vi "Repack Pixels_Pixel Bus to FIFO HSL32x8.vi"(10 "Input Valid":bool=TRUE, 11 "Pixel Bus In":T1={"Pixel Data"={"A"=[0, 0, 0, 0, 0, 0, 0, 0], "R/H"=[0, 0, 0, 0, 0, 0, 0, 0], "G/S"=[0, 0, 0, 0, 0, 0, 0, 0], "B/L"=[0, 0, 0, 0, 0, 0, 0, 0]}, "DV"=[FALSE, FALSE, FALSE, FALSE, FALSE, FALSE, FALSE, FALSE], "EOL"=FALSE, "EOI"=FALSE, "Data Type"=enum."HSL32 x 8"}) -> (2 "Output Valid":bool, 3 "output array":u32[](array[numeric]))   [LabVIEW 2017, in "NI_VDM_FPGA_Basics.lvlib"]
uses:
  <vilib>/visionFPGA/NI_VDM_FPGA_Basics.lvlib
  <vilib>/visionFPGA/Controls/IMAQ FPGA Pixel Bus HSL32x8.ctl
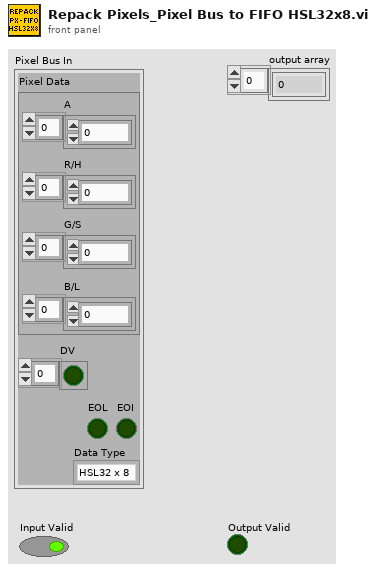
[diagram p1: front panel]
types:
  T1 = typedef "IMAQ FPGA Pixel Bus HSL32x8.ctl" = cluster{"Pixel Data":cluster{"A":u8[], "R/H":u8[], "G/S":u8[], "B/L":u8[]}, "DV":bool[], "EOL":bool, "EOI":bool, "Data Type":enum16{"HSL32 x 8"}}
  T2 = cluster{"A":u8[], "R/H":u8[], "G/S":u8[], "B/L":u8[]}
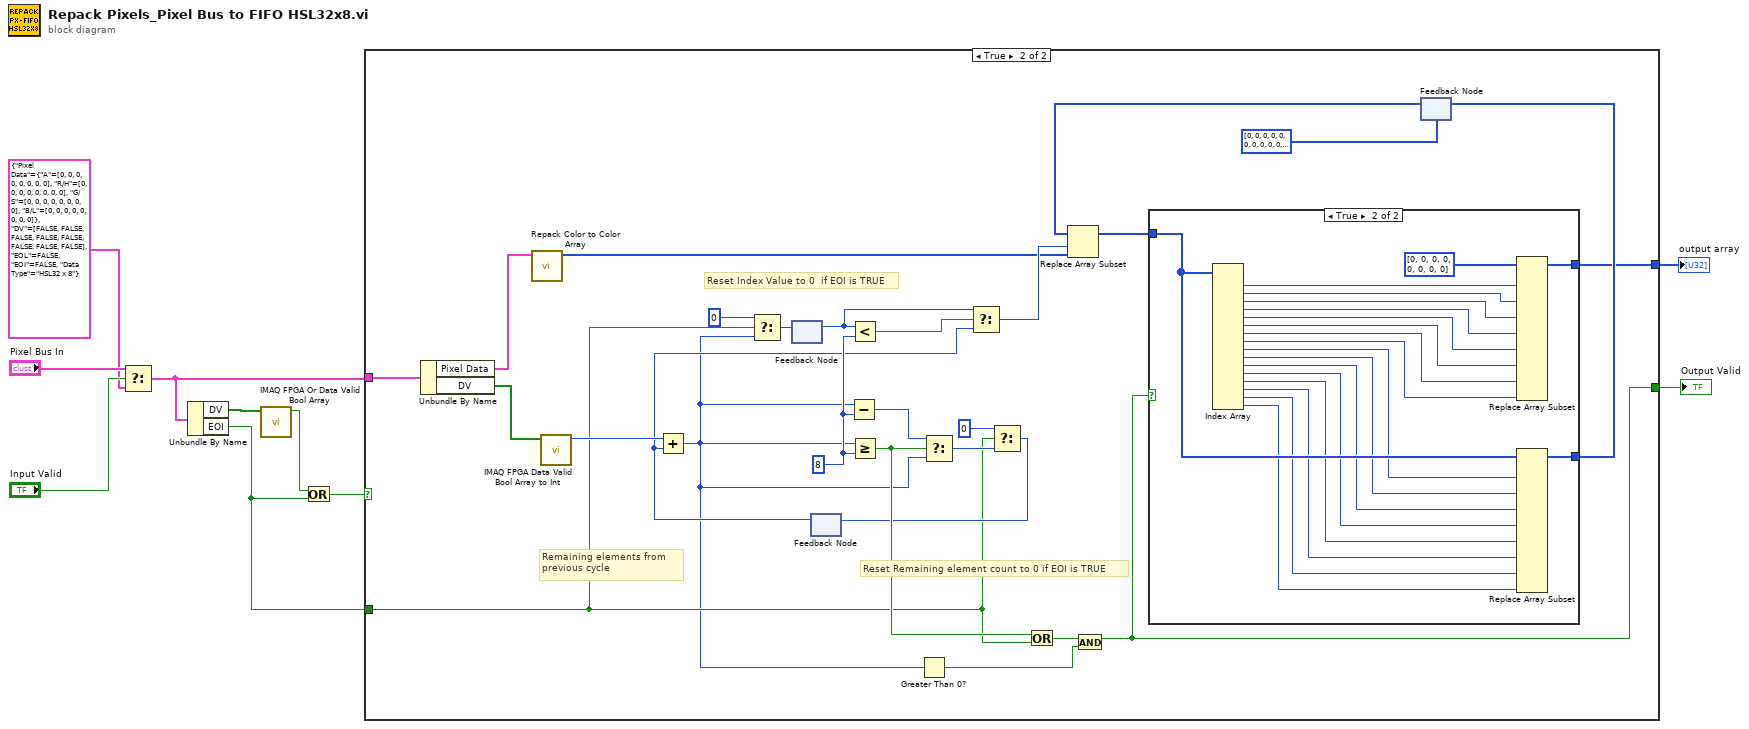
[diagram p0: block diagram]
diagram:
  n1 = Select(t="Pixel Bus In", s="Input Valid", f=T1 {"Pixel Data"={"A"=[0, 0, 0, 0, 0, 0, 0, 0], "R/H"=[0, 0, 0, 0, 0, 0, 0, 0], "G/S"=[0, 0, 0, 0, 0, 0, 0, 0], "B/L"=[0, 0, 0, 0, 0, 0, 0, 0]}, "DV"=[FALSE, FALSE, FALSE, FALSE, FALSE, FALSE, FALSE, FALSE], "EOL"=FALSE, "EOI"=FALSE, "Data Type"=enum."HSL32 x 8"} ("Pixel Bus In")) -> (s? t:f=w5:T1)
  n2 = Unbundle By Name(w5) -> ("DV"=w2:bool[], "EOI"=w4:bool)
  n3 = call <vilib>:"IMAQ FPGA Or Data Valid Bool Array.vi"("DV Array In"=w2) -> ("DV Out"=w1:bool)  [unwired: 10 in]
  n4 = Or(x=w1, y=w4) -> (x .or. y?=w8:bool)
  n5 = case shown="True" w8 {
    tunnel: w5 -> [_ w12]
    tunnel: [_ w33] -> w10
    tunnel: [_ w16] -> w9
    tunnel: w4 -> [_ w17]
    frame False {
    }
    frame True {
      w31 = u16 8 ("y")
      # "Reset Remaining element count to 0 if EOI is TRUE"
      # "Reset Index Value to 0  if EOI is TRUE"
      # "Remaining elements from \nprevious cycle"
      n6 = Unbundle By Name(w12) -> ("Pixel Data"=w11:T2, "DV"=w26:bool[])
      n7 = call <vilib>:"Repack Color to Color Array.vi"("Pixel Data"=w11) -> ("Output array U32x8"=w13:u32[])  [unwired: 10 in]
      n8 = call <vilib>:"IMAQ FPGA Data Valid Bool Array to Int.vi"("DV In"=w26) -> ("Sum DV Out"=w25:u8)  [unwired: 10 in]
      n9 = feedback #1() -> (w30:u16)  [unwired: 1 in]
      n10 = feedback #2() -> (w24:u16)  [unwired: 1 in]
      n11 = Add(x=w25, y=w24) -> (x+y=w15:u16)
      n12 = Select(t=u16 0, s=w17, f=w15) -> (s? t:f=w19:u16)
      n13 = feedback-in #1(w19) -> ()
      n14 = Subtract(x=w15, y=w31) -> (x-y=w32:u16)
      n15 = Less?(x=w30, y=w31) -> (x < y?=w28:bool)
      n16 = Greater Or Equal?(x=w15, y=w31) -> (x >= y?=w27:bool)
      n17 = Greater Than 0?(x=w15) -> (x > 0?=w14:bool)
      n18 = Select(t=w32, s=w27, f=w15) -> (s? t:f=w22:u16)
      n19 = Select(t=w30, s=w28, f=w24) -> (s? t:f=w29:u16)
      n20 = Select(t=u16 0, s=w17, f=w22) -> (s? t:f=w20:u16)
      n21 = feedback-in #2(w20) -> ()
      n22 = Or(x=w27, y=w17) -> (x .or. y?=w23:bool)
      n23 = And(x=w23, y=w14) -> (x .and. y?=w16:bool)
      n24 = feedback #3(u32[] [0, 0, 0, 0, 0, 0, 0, 0, 0, 0, 0, 0, 0, 0, 0, 0] ("Pixel Data")) -> (w35:u32[])
      n25 = Replace Array Subset(array=w35, new element=w13, index=w29) -> (w34:u32[])
      n26 = case shown="True" w16 {
        tunnel: [w38 w58] -> w36
        tunnel: w34 -> [w38 w57]
        tunnel: [_ w39] -> w33
        frame False {
        }
        frame True {
          n27 = Index Array(array=w57) -> (element #1=w55:u32, element #2=w54:u32, element #3=w53:u32, element #4=w52:u32, element #5=w51:u32, element #6=w50:u32, element #7=w49:u32, element #8=w48:u32, element #9=w47:u32, element #10=w46:u32, element #11=w45:u32, element #12=w44:u32, element #13=w43:u32, element #14=w42:u32, element #15=w41:u32, element #16=w40:u32)  [unwired: 16 in]
          n28 = Replace Array Subset(array=u32[] [0, 0, 0, 0, 0, 0, 0, 0] ("Pixel Data"), new element #1=w55, new element #2=w54, new element #3=w53, new element #4=w52, new element #5=w51, new element #6=w50, new element #7=w49, new element #8=w48) -> (w39:u32[])  [unwired: 8 in]
          n29 = Replace Array Subset(array=w57, new element #1=w47, new element #2=w46, new element #3=w45, new element #4=w44, new element #5=w43, new element #6=w42, new element #7=w41, new element #8=w40) -> (w58:u32[])  [unwired: 8 in]
        }
      }
      n30 = feedback-in #3(w36) -> ()
    }
  }
  "output array" <- w10
  "Output Valid" <- w9
